vi "Add Color Ramp.vi"(1 "Limits":cluster{"Low Limit":dbl, "Hi Limit":dbl}[](array[cluster]), 2 "reference in":refnum<vi>) -> (0 "reference out":refnum<vi>)   [LabVIEW 2018]
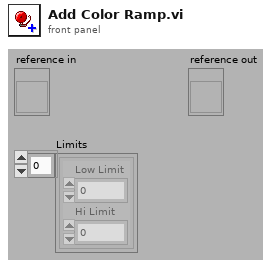
[diagram p1: front panel]
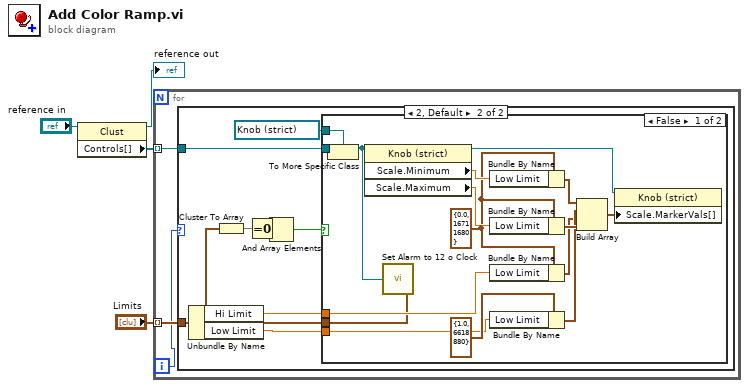
[diagram p0: block diagram]
diagram:
  n1 = property on="Property Node" class="Clust"(reference="reference in") -> (reference out=→"reference out":refnum<vi>, "Controls[]"=w1:refnum<vi>[])  [unwired: 1 in, 1 out]
  n2 = for {
    tunnel: w1 -> [w7] mode=indexing
    tunnel: "Limits" -> [w6] mode=indexing
    i -> [w5]
    n3 = case shown="2, Default" w5 {
      tunnel: w7 -> [_ w15]
      tunnel: w6 -> [_ w9]
      frame 1, 7 {
      }
      frame 2, Default {
        n4 = Unbundle By Name(w9) -> ("Hi Limit"=w12:dbl, "Low Limit"=w13:dbl)
        n5 = Cluster To Array(cluster=w9) -> (array=w11:dbl[])
        n6 = Equal To 0?(x=w11) -> (x = 0?=w10:bool[])
        n7 = And Array Elements(Boolean array=w10) -> (logical AND=w8:bool)
        n8 = case shown="False" w8 {
          tunnel: w15 -> [w23 _]
          tunnel: refnum<vi> refnum ("Knob Refnum") -> [w22 _]
          tunnel: w13 -> [w20 _]
          tunnel: w12 -> [w19 _]
          tunnel: w9 -> [w16 _]
          frame False {
            w18 = cluster{"Low Limit":dbl, u32} {"Low Limit"=0.0, 16711680}
            n9 = To More Specific Class(target class=w22, reference=w23) -> (specific class reference=w17:refnum<vi>)  [unwired: 1 in, 1 out]
            n10 = property on="Property Node" class="Knob (strict)"(reference=w17) -> (reference out=w21:refnum<vi>, "Scale.Minimum"=w29:dbl, "Scale.Maximum"=w31:dbl)  [unwired: 1 in, 1 out]
            n11 = call "Set Alarm to 12 o Clock.vi"("Limits"=w16, "Knob Refnum"=w17) -> ()
            n12 = Bundle By Name(cluster=w18, "Low Limit"=w29) -> (w27:cluster{"Low Limit":dbl, u32})
            n13 = Bundle By Name(cluster=w18, "Low Limit"=w31) -> (w30:cluster{"Low Limit":dbl, u32})
            n14 = Bundle By Name(cluster=w18, "Low Limit"=w19) -> (w25:cluster{"Low Limit":dbl, u32})
            n15 = Bundle By Name(cluster=cluster{"Low Limit":dbl, u32} {"Low Limit"=1.0, 6618880}, "Low Limit"=w20) -> (w26:cluster{"Low Limit":dbl, u32})
            n16 = Build Array(w27, w26, w25, w30) -> (w28:cluster{"Low Limit":dbl, u32}[])
            n17 = property on="Property Node" class="Knob (strict)"(reference=w21, "Scale.MarkerVals[]"=w28) -> ()  [unwired: 1 in, 2 out]
          }
          frame True {
          }
        }
      }
    }
  }
